vi "Acquire IQ _GESys.vi"(6 "timeout (10 sec)":dbl=60.0 format="%#_13g", 7 "Carrier Frequency (Hz)":dbl=902200000.0 format="%#.3p", 8 "error in (no error)":errorcluster, 9 "Reference Position (%)":dbl=5.0, 10 "Burst Length (sec)":dbl=0.35, 11 "instrument handle":refnum<k15>) -> (0 "error out":errorcluster, 1 "IQ":cluster{"t0":dbl, "dt":dbl, "Y":cdb[]} caption="data" {"Y" format="%_2g"}, 2 "Pre-Trigger":dbl, 3 "instrument handle out":refnum<k15>)   [LabVIEW 2018]
uses:
  <instrlib>/niRFSA/niRFSA.llb/niRFSA Acquisition Types.ctl
  <instrlib>/niRFSA/niRFSA.llb/niRFSA Configure IQ Power Edge Ref Trigger.vi
  <instrlib>/niRFSA/niRFSA.llb/niRFSA Fetch IQ (Complex Cluster 1Rec 1Chan).vi
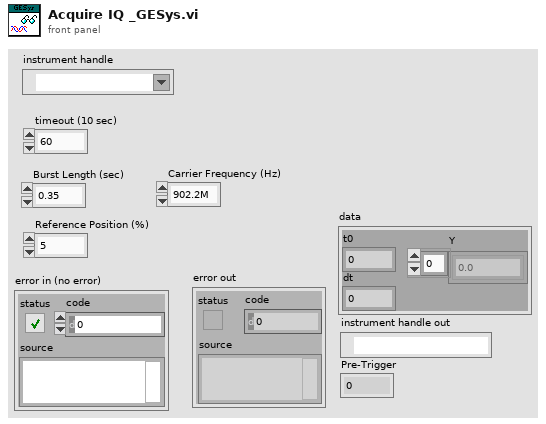
[diagram p1: front panel]
types:
  T1 = typedef "niRFSA Acquisition Types.ctl" = i32
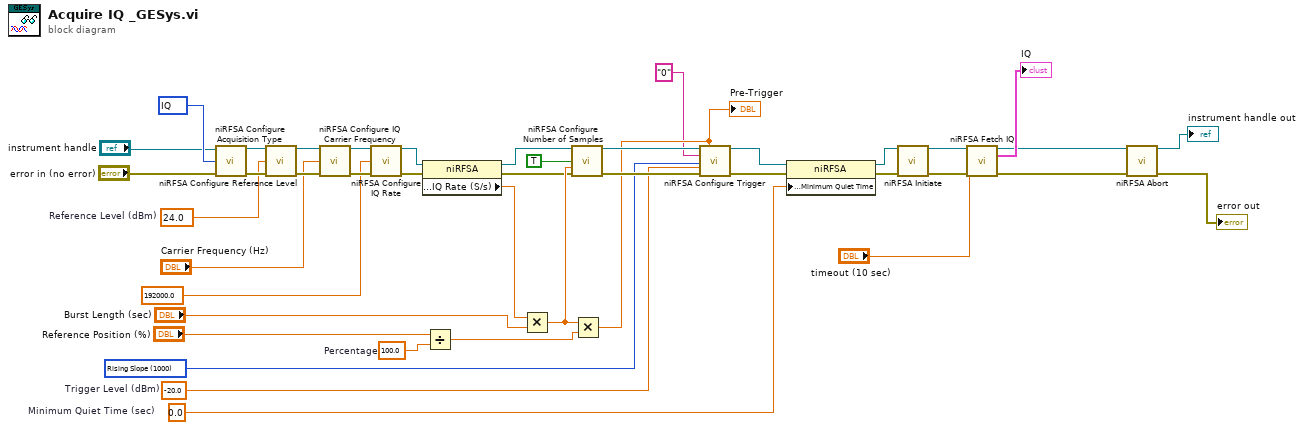
[diagram p0: block diagram]
diagram:
  w24 = 0.0  # Minimum Quiet Time (sec)
  w30 = -20.0  # Trigger Level (dBm)
  w12 = 1000 items=["Rising Slope"=1000, "Falling Slope"=1001] ("Trigger Slope")
  w33 = 24.0  # Reference Level (dBm)
  w18 = 100.0  # Percentage
  w34 = T1 100 items=["IQ"=100, "Spectrum"=101] ("acquisition type")
  n1 = call <instrlib>:"niRFSA Configure Acquisition Type.vi"("instrument handle"="instrument handle", "acquisition type"=w34, "error in"="error in (no error)") -> ("instrument handle out"=w37:refnum<k15>, "error out"=w38:errorcluster)  [unwired: 11 in]
  n2 = call <instrlib>:"niRFSA Configure Reference Level.vi"("instrument handle"=w37, "reference level (dBm)"=w33, "error in"=w38) -> ("instrument handle out"=w42:refnum<k15>, "error out"=w41:errorcluster)  [unwired: 11 in]
  n3 = call <instrlib>:"niRFSA Configure IQ Carrier Frequency.vi"("instrument handle"=w42, "carrier frequency"="Carrier Frequency (Hz)", "error in"=w41) -> ("instrument handle out"=w36:refnum<k15>, "error out"=w35:errorcluster)  [unwired: 11 in]
  n4 = call <instrlib>:"niRFSA Configure IQ Rate.vi"("instrument handle"=w36, "IQ rate (S/s)"=192000.0 ("IQ Rate (S/s)"), "error in"=w35) -> ("instrument handle out"=w16:refnum<k15>, "error out"=w17:errorcluster)  [unwired: 11 in]
  n5 = property class="niRFSA"(reference=w16, error in=w17) -> (reference out=w14:refnum<k15>, error out=w15:errorcluster, "Acquisition:IQ:IQ Rate (S/s)"=w13:dbl)
  n6 = Divide(x="Reference Position (%)", y=w18) -> (x/y=w20:dbl)
  n7 = Multiply(x=w13, y="Burst Length (sec)") -> (x*y=w28:dbl)
  n8 = call <instrlib>:"niRFSA Configure Number of Samples.vi"("instrument handle"=w14, "number of samples is finite"=TRUE, "samples per record"=w28, "error in"=w15) -> ("instrument handle out"=w40:refnum<k15>, "error out"=w39:errorcluster)  [unwired: 10 in]
  n9 = Multiply(x=w28, y=w20) -> (x*y=w27:dbl)
  "Pre-Trigger" <- w27
  n10 = call-poly <instrlib>:"niRFSA Configure Trigger.vi"("instrument handle"=w40, "pretrigger samples"=w27, "source"="0", "slope"=w12, "level"=w30, "error in"=w39) -> ("instrument handle out"=w26:refnum<k15>, "error out"=w25:errorcluster)  [unwired: 8 in]
  n11 = property class="niRFSA"(reference=w26, error in=w25, "Triggers:Ref:Minimum Quiet Time"=w24) -> (reference out=w23:refnum<k15>, error out=w22:errorcluster)
  n12 = call <instrlib>:"niRFSA Initiate.vi"("instrument handle"=w23, "error in"=w22) -> ("instrument handle out"=w10:refnum<k15>, "error out"=w9:errorcluster)  [unwired: 12 in]
  n13 = call-poly <instrlib>:"niRFSA Fetch IQ.vi"("instrument handle"=w10, "timeout (10 sec)"="timeout (10 sec)", "error in"=w9) -> ("instrument handle out"=w4:refnum<k15>, "data"=→"IQ":cluster{"t0":dbl, "dt":dbl, "Y":cdb[]}, "error out"=w3:errorcluster)  [unwired: 10 in]
  n14 = call <instrlib>:"niRFSA Abort.vi"("instrument handle"=w4, "error in"=w3) -> ("instrument handle out"=→"instrument handle out":refnum<k15>, "error out"=→"error out":errorcluster)  [unwired: 12 in]
